vi "MccHat_init.vi"(7 "commands":string[](array[string])=["init-boards", "set-tc-type 0 all T", "set-input-range 1 5V", "enable-channel 0 0,3", "enable-channel 1 0-7"], 8 "error in":errorcluster, 10 "port":u16, 11 "address":string) -> (0 "error out":errorcluster, 3 "conn_id":refnum<k5>, 4 "status":bool, 5 "server":string)   [LabVIEW 2019]
panel:
  out "status_each":bool[](array[boolean])
  out "msg_each":string[](array[string])
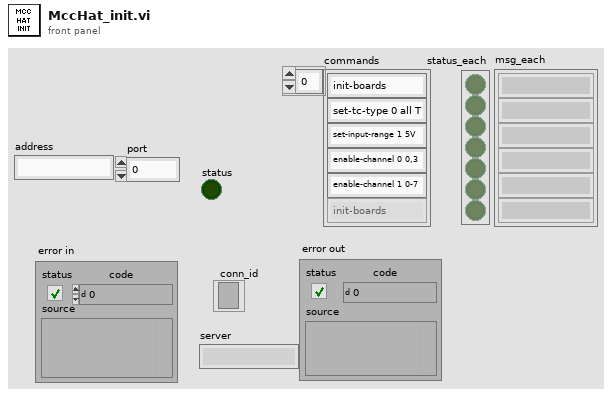
[diagram p1: front panel]
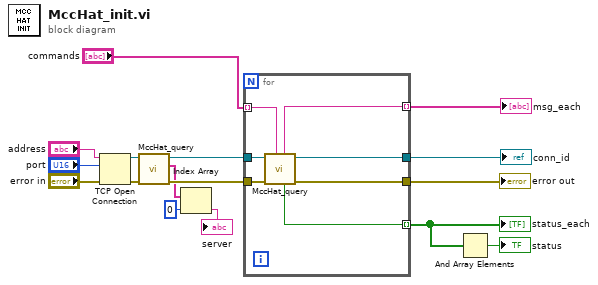
[diagram p0: block diagram]
diagram:
  n1 = TCP Open Connection(address="address", remote port or service name="port", error in (no error)="error in") -> (connection ID=w7:refnum<k5>, error out=w5:errorcluster)  [unwired: 2 in]
  n2 = call "MccHat_query.vi"("error in"=w5, "conn_id_in"=w7) -> ("error out"=w4:errorcluster, "string_array"=w3:string[], "conn_id_out"=w6:refnum<k5>)  [unwired: 5 in, 2 out]
  n3 = Index Array(array=w3, index=0) -> (element=→"server":string)
  n4 = for {
    tunnel: w4 -> [w23]
    tunnel: w6 -> [w22]
    tunnel: [w21] -> w11 mode=indexing
    tunnel: "commands" -> [w20] mode=indexing
    tunnel: [w19] -> w12 mode=indexing
    tunnel: [w18] -> w9
    tunnel: [w17] -> w8
    n5 = call "MccHat_query.vi"("command"=w20, "error in"=w23, "conn_id_in"=w22) -> ("error out"=w18:errorcluster, "conn_id_out"=w17:refnum<k5>, "status"=w21:bool, "string_raw"=w19:string)  [unwired: 4 in, 1 out]
  }
  "error out" <- w9
  "msg_each" <- w12
  "conn_id" <- w8
  "status_each" <- w11
  n6 = And Array Elements(Boolean array=w11) -> (logical AND=→"status":bool)
